vi "prueba4_21241028_ElminMejia.vi"() -> ()   [LabVIEW 2011]
uses:
  Controlprueba4_21241028 _ElminMejia.ctl
panel:
  out "Array":T1(array[cluster]) {"tanque4" scale=0.0..50.0; "tanque3" scale=0.0..50.0; "tanque2" scale=0.0..50.0; "tanque1" scale=0.0..50.0}
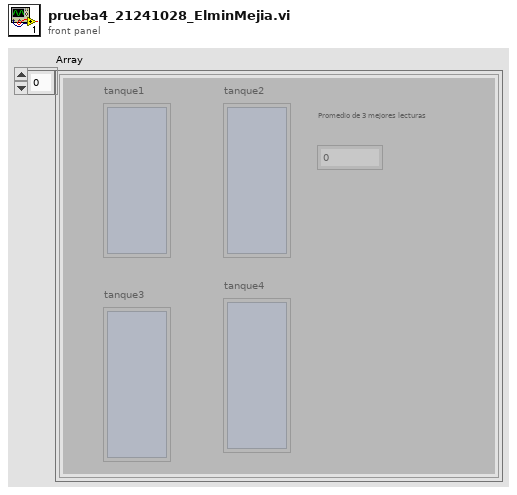
[diagram p1: front panel]
types:
  T1 = cluster{"tanque1":i32, "tanque2":i32, "tanque3":i32, "tanque4":i32, "Promedio de 3 mejores lecturas":dbl}[]
  T2 = typedef "Controlprueba4_21241028 _ElminMejia.ctl" = enum16{"Inicializar variables", "Rellenar tanques", "Promedio 3 mejores lects", "Finalizar"}
  T3 = cluster{"tanque1":i32, "tanque2":i32, "tanque3":i32, "tanque4":i32, "Promedio de 3 mejores lecturas":dbl}
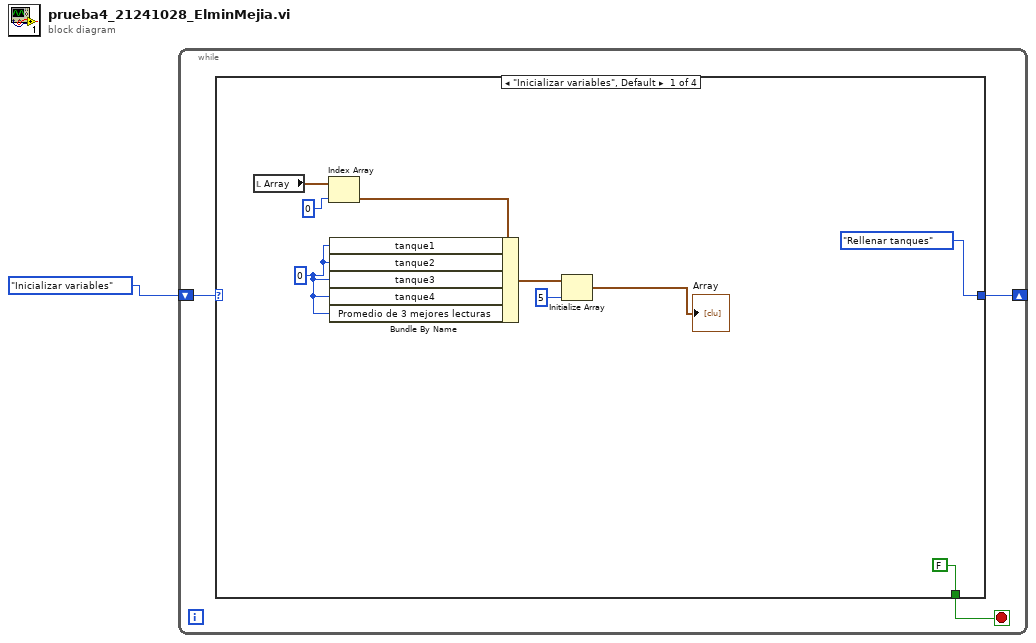
[diagram p0: block diagram]
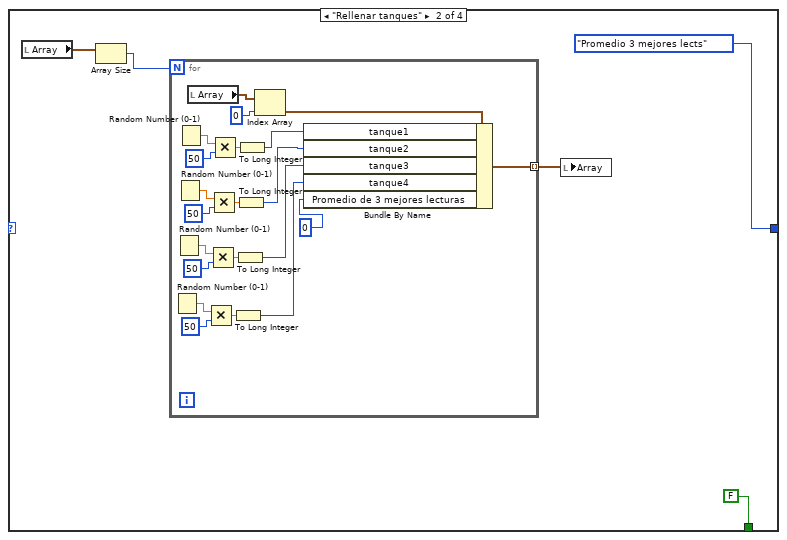
[diagram p2: hidden frame]
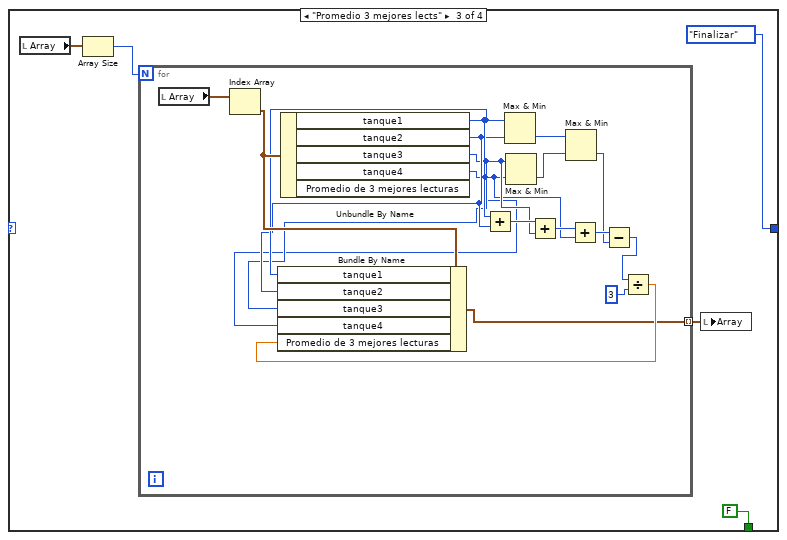
[diagram p3: hidden frame]
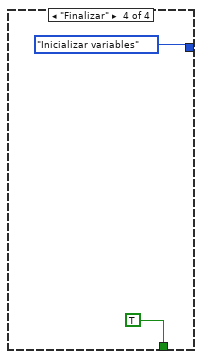
[diagram p4: hidden frame]
diagram:
  n1 = while {
    shift-right: [w3] -> _
    shift-left: Controlprueba4_21241028__ElminMejia."Inicializar variables" -> [w4]
    stop <- w2 stop-if-true
    n2 = case shown="\"Inicializar variables\", Default" w4 {
      tunnel: [Controlprueba4_21241028__ElminMejia."Rellenar tanques" Controlprueba4_21241028__ElminMejia."Promedio 3 mejores lects" Controlprueba4_21241028__ElminMejia."Finalizar" Controlprueba4_21241028__ElminMejia."Inicializar variables"] -> w3
      tunnel: [FALSE FALSE FALSE TRUE] -> w2
      frame "Inicializar variables", Default {
        w9 = 0
        n3 = local read "Array"() -> (w11:T1)
        n4 = Index Array "Index Array"(array=w11, index=0) -> (element=w10:T3)
        n5 = Bundle By Name(cluster=w10, "tanque1"=w9, "tanque2"=w9, "tanque3"=w9, "tanque4"=w9, "Promedio de 3 mejores lecturas"=w9) -> (w7:T3)
        n6 = Initialize Array "Initialize Array"(w7, 5) -> (→"Array":T1)
      }
      frame "Rellenar tanques" {
        n7 = local read "Array"() -> (w16:T1)
        n8 = Array Size(array=w16) -> (size(s)=w15:i32)
        n9 = for {
          N: w15 -> [_]
          tunnel: [w19] -> w14 mode=indexing
          n10 = Random Number (0-1)() -> (number: 0 to 1=w25:dbl)
          n11 = Random Number (0-1)() -> (number: 0 to 1=w28:dbl)
          n12 = Random Number (0-1)() -> (number: 0 to 1=w31:dbl)
          n13 = Random Number (0-1)() -> (number: 0 to 1=w35:dbl)
          n14 = local read "Array"() -> (w39:T1)
          n15 = Multiply(x=w25, y=50) -> (x*y=w26:dbl)
          n16 = Multiply(x=w28, y=50) -> (x*y=w27:dbl)
          n17 = Multiply(x=w31, y=50) -> (x*y=w32:dbl)
          n18 = Multiply(x=w35, y=50) -> (x*y=w34:dbl)
          n19 = To Long Integer(number=w26) -> (32bit integer=w21:i32)
          n20 = To Long Integer(number=w27) -> (32bit integer=w22:i32)
          n21 = To Long Integer(number=w32) -> (32bit integer=w23:i32)
          n22 = To Long Integer(number=w34) -> (32bit integer=w33:i32)
          n23 = Index Array "Index Array"(array=w39, index=0) -> (element=w37:T3)
          n24 = Bundle By Name(cluster=w37, "tanque1"=w33, "tanque2"=w23, "tanque3"=w22, "tanque4"=w21, "Promedio de 3 mejores lecturas"=0) -> (w19:T3)
        }
        n25 = local write "Array"(w14) -> ()
      }
      frame "Promedio 3 mejores lects" {
        n26 = local read "Array"() -> (w44:T1)
        n27 = Array Size(array=w44) -> (size(s)=w43:i32)
        n28 = for {
          N: w43 -> [_]
          tunnel: [w45] -> w40 mode=indexing
          n29 = local read "Array"() -> (w60:T1)
          n30 = Index Array "Index Array"(array=w60) -> (element=w51:T3)  [unwired: 1 in]
          n31 = Unbundle By Name(w51) -> ("tanque1"=w50:i32, "tanque2"=w49:i32, "tanque3"=w48:i32, "tanque4"=w47:i32)  [unwired: 1 out]
          n32 = Add(x=w50, y=w49) -> (x+y=w57:i32)
          n33 = Max & Min(x=w50, y=w49) -> (min(x,y)=w59:i32)  [unwired: 1 out]
          n34 = Max & Min(x=w48, y=w47) -> (min(x,y)=w58:i32)  [unwired: 1 out]
          n35 = Add(x=w57, y=w48) -> (x+y=w56:i32)
          n36 = Max & Min(x=w59, y=w58) -> (min(x,y)=w54:i32)  [unwired: 1 out]
          n37 = Add(x=w56, y=w47) -> (x+y=w55:i32)
          n38 = Subtract(x=w55, y=w54) -> (x-y=w53:i32)
          n39 = Divide(x=w53, y=3) -> (x/y=w46:dbl)
          n40 = Bundle By Name(cluster=w51, "tanque1"=w50, "tanque2"=w49, "tanque3"=w48, "tanque4"=w47, "Promedio de 3 mejores lecturas"=w46) -> (w45:T3)
        }
        n41 = local write "Array"(w40) -> ()
      }
      frame "Finalizar" {
      }
    }
  }
